vi "timer vi.vi"() -> ()   [LabVIEW 2018]
panel:
  out "Array 2":dbl[](array[numeric])
  out "Array":dbl[](array[numeric])
  out "Time 2":u32
  out "Time 1":u32
  in  "Iterations":i32=100000
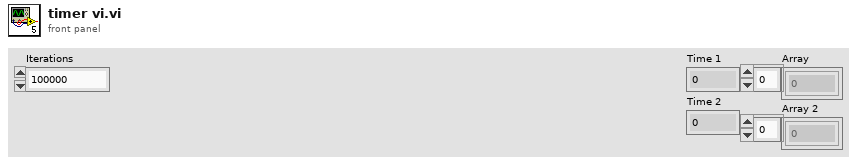
[diagram p1: front panel]
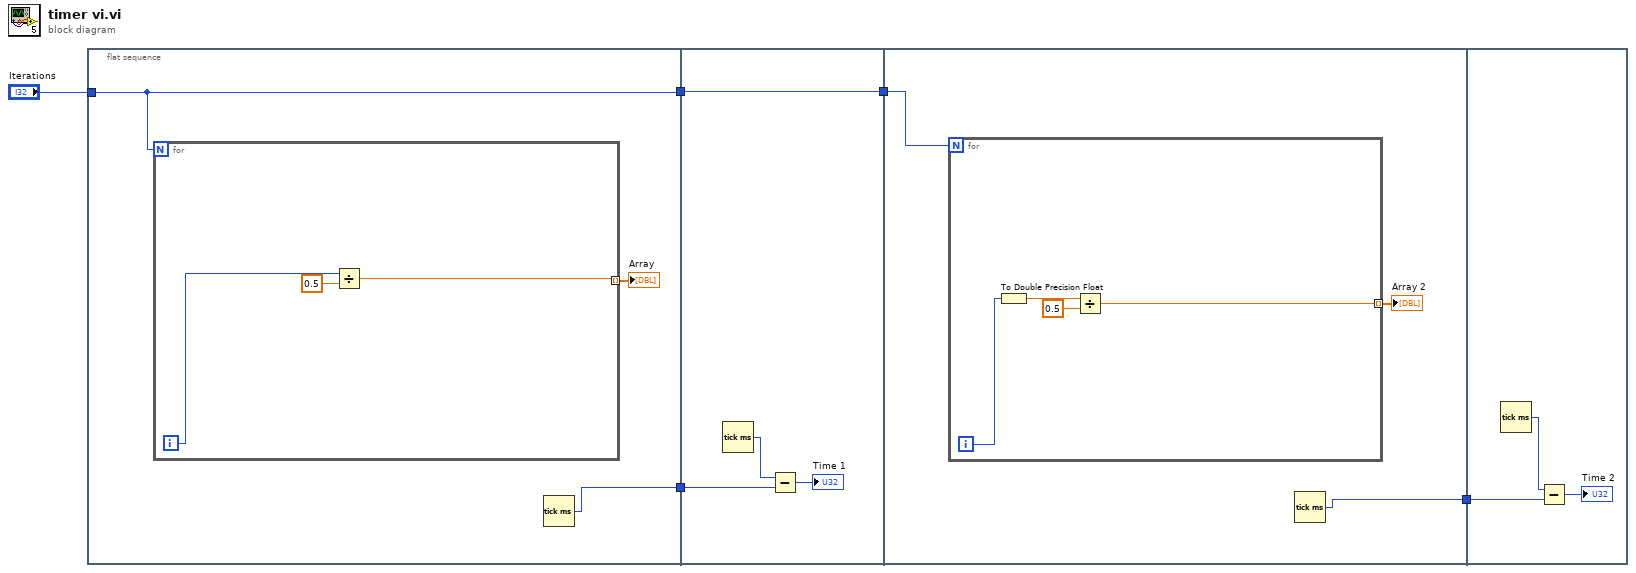
[diagram p0: block diagram]
diagram:
  n1 = flat-sequence {
    tunnel: [w7] -> w4
    tunnel: [w8] -> w3
    tunnel: "Iterations" -> [w7]
    tunnel: [w15] -> w5
    tunnel: w4 -> [w15]
    tunnel: w3 -> [w13]
    tunnel: w5 -> [w18]
    tunnel: [w17] -> w2
    tunnel: w2 -> [w25]
    frame #0 {
      n2 = for {
        N: w7 -> [_]
        tunnel: [w9] -> w6 mode=indexing
        i -> [w11]
        n3 = Divide(x=w11, y=0.5) -> (x/y=w9:dbl)
      }
      "Array" <- w6
      n4 = Tick Count (ms)() -> (millisecond timer value=w8:u32)
    }
    frame #1 {
      n5 = Tick Count (ms)() -> (millisecond timer value=w14:u32)
      n6 = Subtract(x=w14, y=w13) -> (x-y=→"Time 1":u32)
    }
    frame #2 {
      n7 = for {
        N: w18 -> [_]
        tunnel: [w19] -> w16 mode=indexing
        i -> [w22]
        n8 = To Double Precision Float(number=w22) -> (double precision float=w21:dbl)
        n9 = Divide(x=w21, y=0.5) -> (x/y=w19:dbl)
      }
      "Array 2" <- w16
      n10 = Tick Count (ms)() -> (millisecond timer value=w17:u32)
    }
    frame #3 {
      n11 = Tick Count (ms)() -> (millisecond timer value=w24:u32)
      n12 = Subtract(x=w24, y=w25) -> (x-y=→"Time 2":u32)
    }
  }
